vi "append_raw_data.vi"(8 "error in (no error)":errorcluster, 10 "channels raw data block":T1, 11 "GenericDAQ in":refnum<class "GenericDAQ.lvclass">) -> (0 "error out":errorcluster, 3 "GenericDAQ out":refnum<class "GenericDAQ.lvclass">)   [LabVIEW 2010, in "GenericDAQ.lvclass"]
doc: "Appends data block to software buffer."
uses:
  GenericDAQ.lvclass
  common/arrays/pixel_raw_data_array.ctl
  GenericDAQ.lvclass/GenericDAQ.ctl
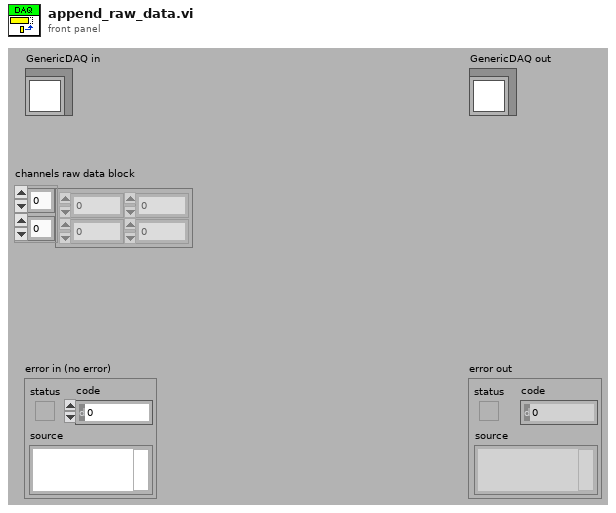
[diagram p1: front panel]
types:
  T1 = typedef "pixel_raw_data_array.ctl" = dbl[][]
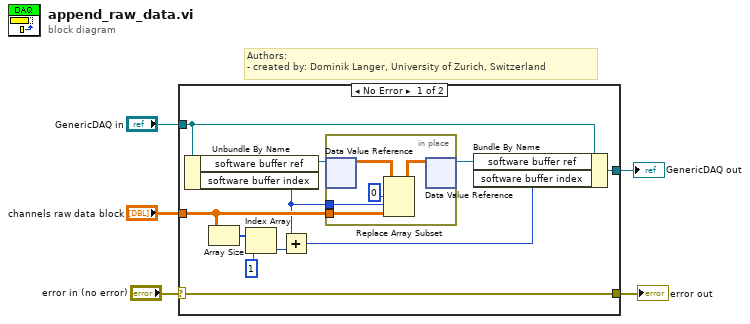
[diagram p0: block diagram]
diagram:
  # "Authors: \n- created by: Dominik Langer, University of Zurich, Switzerland"
  n1 = case shown="No Error" "error in (no error)" {
    selector: "error in (no error)" -> [w16 w23]
    tunnel: [w16 w23] -> w4
    tunnel: [w12 w22] -> w2
    tunnel: "GenericDAQ in" -> [w13 w22]
    tunnel: "channels raw data block" -> [w11 _]
    frame No Error {
      n2 = Unbundle By Name(w13) -> ("software buffer ref"=w15:refnum<data-value>, "software buffer index"=w7:i32)
      n3 = Array Size(array=w11) -> (size(s)=w10:i32[])
      n4 = Index Array(array=w10, index=1) -> (element=w8:i32)
      n5 = Add(x=w7, y=w8) -> (x+y=w6:i32)
      n6 = in-place {
        in-place-border: w11 -> [w21]
        in-place-border: w7 -> [w18]
        n7 = in-place-dvr #1(w15) -> (w20:T1)  [unwired: 1 out]
        n8 = Replace Array Subset(array=w20, new element=w21, index (row)=0 ("disabled index (row)"), index (col)=w18) -> (w19:T1)
        n9 = in-place-dvr #1(w19) -> (w14:refnum<data-value>)  [unwired: 1 out]
      }
      n10 = Bundle By Name(cluster=w13, "software buffer ref"=w14, "software buffer index"=w6) -> (w12:refnum<class "GenericDAQ.lvclass">)
    }
    frame Error {
    }
  }
  "error out" <- w4
  "GenericDAQ out" <- w2
